vi "Encode repeated bytes.vi"(7 "Field Number":i32, 10 "bytes":cluster{"bytes":u8[]}[](array[cluster]) {"bytes" format="%.0x"}, 11 "Buffer in":u8[](array[numeric]) format="%.0x") -> (3 "Buffer":u8[](array[numeric]) format="%.0x")   [LabVIEW 2020, in "LV-Proto.lvlib"]
uses:
  LV-Proto.lvlib
  Wire Encode Tag.vi
  Wire Encode Varint I32.vi
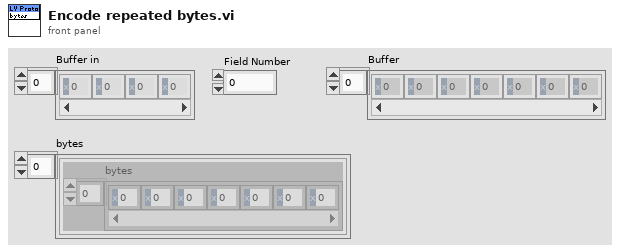
[diagram p1: front panel]
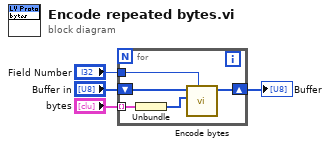
[diagram p0: block diagram]
diagram:
  n1 = for {
    shift-right: [w5] -> w3
    shift-left: "Buffer in" -> [w8]
    tunnel: "Field Number" -> [w6]
    tunnel: "bytes" -> [w9] mode=indexing
    n2 = Unbundle(w9) -> ("bytes"=w7:u8[])
    n3 = call "Encode bytes.vi"("Field Number"=w6, "bytes"=w7, "Buffer in"=w8) -> ("Buffer"=w5:u8[])  [unwired: 8 in]
  }
  "Buffer" <- w3
